vi "Read Double.vi"(11 "Event in":refnum<class "Event Double.lvclass">) -> (2 "Double":dbl, 3 "Event out":refnum<class "Event Double.lvclass">)   [LabVIEW 2016, in "Event Source.lvlib" / "Event Double.lvclass"]
uses:
  Event Double.lvclass
  Event Double.lvclass/Event Double.ctl
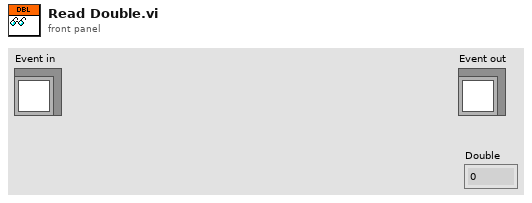
[diagram p1: front panel]
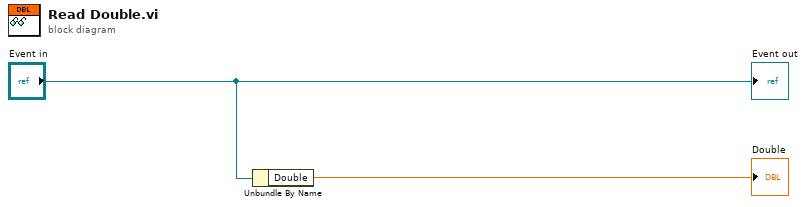
[diagram p0: block diagram]
diagram:
  n1 = Unbundle By Name("Event in") -> ("Double"=→"Double":dbl)
  "Event out" <- "Event in"
